vi "ccidinfo-w.vi"(1 "Data":string, 2 "Data Type":T1, 3 "Slot":T2) -> ()   [LabVIEW 2013]
uses:
  SystemCode/SysControl/Slot.ctl
  CCID info.ctl
  GlobalValue.vi
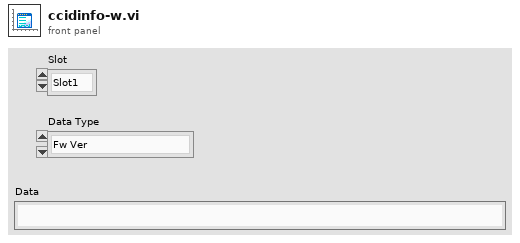
[diagram p1: front panel]
types:
  T1 = typedef "CCID info.ctl" = enum16{"Fw Ver", "HW Ver", "CCID", "WiFiName", "DevID"}
  T2 = typedef "Slot.ctl" = enum16{"Slot1", "Slot2", "Slot3", "Slot4"}
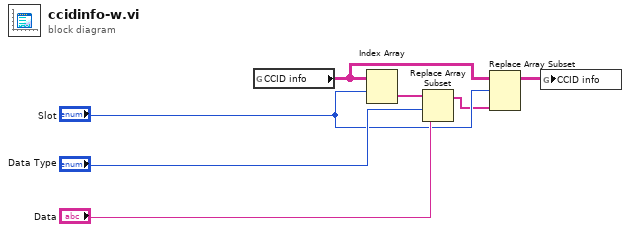
[diagram p0: block diagram]
diagram:
  n1 = global read "GlobalValue.vi" "CCID info"() -> (w3:string[][])
  n2 = Index Array(array=w3, index (row)="Slot") -> (element=w4:string[])  [unwired: 1 in]
  n3 = Replace Array Subset(array=w4, new element="Data", index="Data Type") -> (w2:string[])
  n4 = Replace Array Subset(array=w3, new element=w2, index (row)="Slot") -> (w1:string[][])  [unwired: 1 in]
  n5 = global write "GlobalValue.vi" "CCID info"(w1) -> ()
